vi "poly_global_eco_minus.vi"(4 "code (w/ ECO)":i32) -> (1 "code (- ECO)":i32)   [LabVIEW 2015]
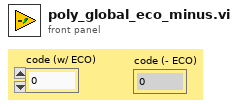
[diagram p1: front panel]
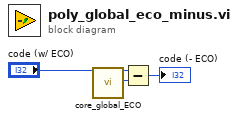
[diagram p0: block diagram]
diagram:
  n1 = call "core_global_ECO.vi"() -> ("LVutils global ECO"=w1:i32)
  n2 = Subtract(x="code (w/ ECO)", y=w1) -> (x-y=→"code (- ECO)":i32)
